vi "test_av_ljud.vi"() -> ()   [LabVIEW 2015]
uses:
  <vilib>/express/express analysis/Spectral/Block/exnSpectralBlock spectral measurements peak poly.vi
  <vilib>/express/express analysis/Spectral/Block/exnSpectralBlock spectral measurements peak array WFM.vi
  <vilib>/express/express analysis/Spectral/XNode/ExpressSpectralMeasurementsBlockNode.xnode
panel:
  out "Time-Domain":waveform(dbl)[](graph)
  out "Spectrum":cluster{"f0":dbl, "df":dbl, "magnitude":dbl[]}[](graph)
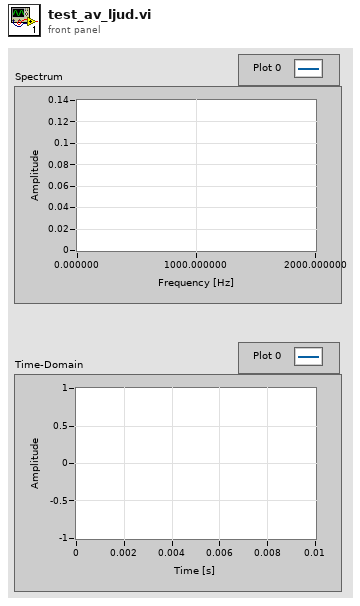
[diagram p1: front panel]
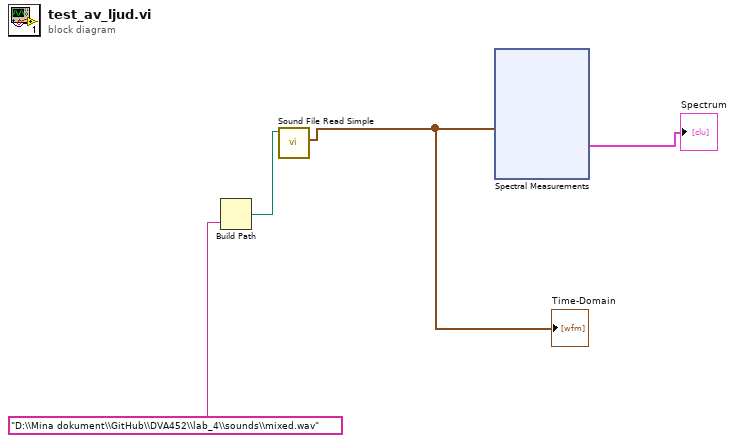
[diagram p0: block diagram]
diagram:
  n1 = Build Path(name or relative path="D:\\Mina dokument\\GitHub\\DVA452\\lab_4\\sounds\\mixed.wav") -> (appended path=w2:path)  [unwired: 1 in]
  n2 = call <vilib>:"Sound File Read Simple.vi"("path"=w2) -> ("data"=w1:waveform(dbl)[])  [unwired: 7 in, 3 out]
  "Time-Domain" <- w1
  n3 = xnode "Spectral Measurements"("Signals"=w1) -> ("FFT - (Peak)"=→"Spectrum":cluster{"f0":dbl, "df":dbl, "magnitude":dbl[]}[])  [unwired: 1 in, 2 out]
